vi "Bitwise XOR (Greyscale).vi"(8 "error in (no error)":errorcluster, 9 "Greyscale Image Destination":T1, 10 "Greyscale Image B":T1, 11 "Greyscale Image A":T1) -> (0 "error out":errorcluster, 3 "Greyscale Image Destination (duplicate)":T1)   [LabVIEW 2020, in "g_ar_toolkit.image.lvlib"]
uses:
  g_ar_toolkit.image.lvlib
  Greyscale Image.ctl
  BitwiseOperation.ctl
  253e84a8-32ce-4670-ae81-0d341c439dd3.vi
  g_ar_toolkit.common/Module Path.vi
  <vilib>/Utility/error.llb/Error Cluster From Error Code.vi
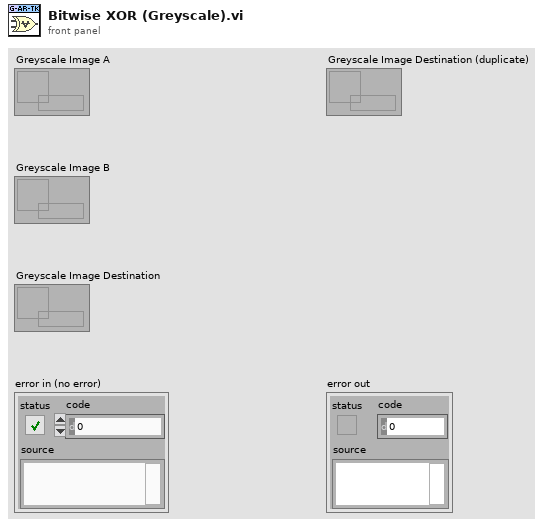
[diagram p1: front panel]
types:
  T1 = typedef "g_ar_toolkit.image.lvlib/Greyscale Image.ctl" = refnum<data-value>
  T2 = typedef "g_ar_toolkit.image.lvlib/BitwiseOperation.ctl" = enum8{"OR", "AND", "XOR"}
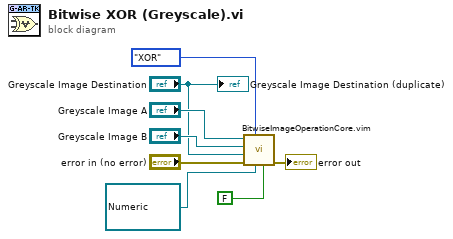
[diagram p0: block diagram]
diagram:
  n1 = call "BitwiseImageOperationCore.vim"("HasMask"=FALSE, "Mask"=refnum<data-value> refnum, "BitwiseOperation"=BitwiseOperation."XOR", "error in (no error)"="error in (no error)", "Destination Image"="Greyscale Image Destination", "Image B"="Greyscale Image B", "Image A"="Greyscale Image A") -> ("error out"=→"error out":errorcluster)  [unwired: 4 in]
  "Greyscale Image Destination (duplicate)" <- "Greyscale Image Destination"
